vi "User.Init.vi"(8 "error in (no error)":errorcluster) -> (0 "error out":errorcluster)   [LabVIEW 2013]
uses:
  User.Level.ctl
  Global/ApplicationGlobal.vi
  User.Global.vi
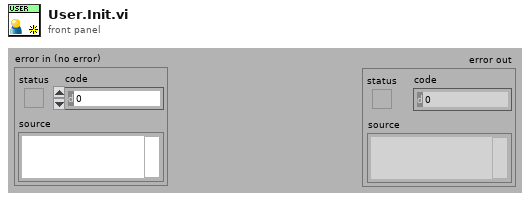
[diagram p1: front panel]
types:
  T1 = enum32{"invalid app kind", "Development System", "Run Time System", "Student Edition", "Embedded LabVIEW", "Evaluation", "Custom"}
  T2 = typedef "User.Level.ctl" = enum16{"-", "Operator", "Technician", "Administrator"}
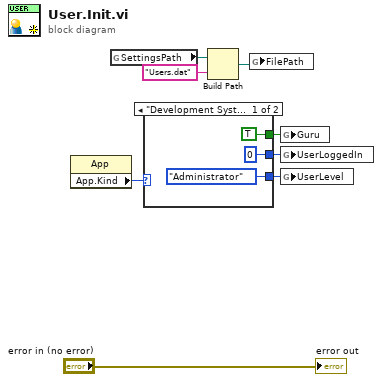
[diagram p0: block diagram]
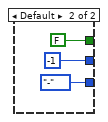
[diagram p2: hidden frame]
diagram:
  n1 = property class="App"() -> ("App.Kind"=w1:T1)  [unwired: 2 in, 2 out]
  n2 = global read "ApplicationGlobal.vi" "SettingsPath"() -> (w8:path)
  n3 = case shown="\"Development System\"" w1 {
    tunnel: [TRUE ("Guru") FALSE ("Guru")] -> w4
    tunnel: [0 ("UserLoggedIn") -1 ("UserLoggedIn")] -> w3
    tunnel: [User.Level."Administrator" ("UserLevel") User.Level."-" ("UserLevel")] -> w2
    frame "Development System" {
    }
    frame Default {
    }
  }
  n4 = Build Path(base path=w8, name or relative path="Users.dat") -> (appended path=w6:path)
  n5 = global write "User.Global.vi" "FilePath"(w6) -> ()
  n6 = global write "User.Global.vi" "Guru"(w4) -> ()
  n7 = global write "User.Global.vi" "UserLoggedIn"(w3) -> ()
  n8 = global write "User.Global.vi" "UserLevel"(w2) -> ()
  "error out" <- "error in (no error)"
